vi "SV Time Waveforms State Manager.vi"(6 "delete hit index (-1 = last)":i32=-1, 7 "action":u16(ring)=3 items=["Initialize to Empty", "Add to State", "Delete from State", "Get Identifiers", "Get State"], 9 "1D Array of Current Time Data\n[reference, response0..N]":waveform(dbl)[](array[waveform]), 10 "Array of Node IDentifiers\n[reference{node, dir}, response0{node, dir}, ...]":T2(array[cluster]) {"active node" format="%04.0f"}, 11 "Time-Domain State":T3 {"IDentifiers"."Array of Node IDentifiers[reference{node, dir}, response0{node, dir}, ...]"."active node" format="%04.0f"}) -> (1 "2D Array of Time Data\n[[reference, response0..N] by [hit0..K]]":waveform(dbl)[][](array[waveform]), 2 "IDentifiers":T1(array[cluster]) {"Array of Node IDentifiers[reference{node, dir}, response0{node, dir}, ...]"."active node" format="%04.0f"}, 3 "Time-Domain State out":T3 {"IDentifiers"."Array of Node IDentifiers[reference{node, dir}, response0{node, dir}, ...]"."active node" format="%04.0f"}, 4 "number of impacts":i32[](array[numeric]), 5 "state changed":bool)   [LabVIEW 2017]
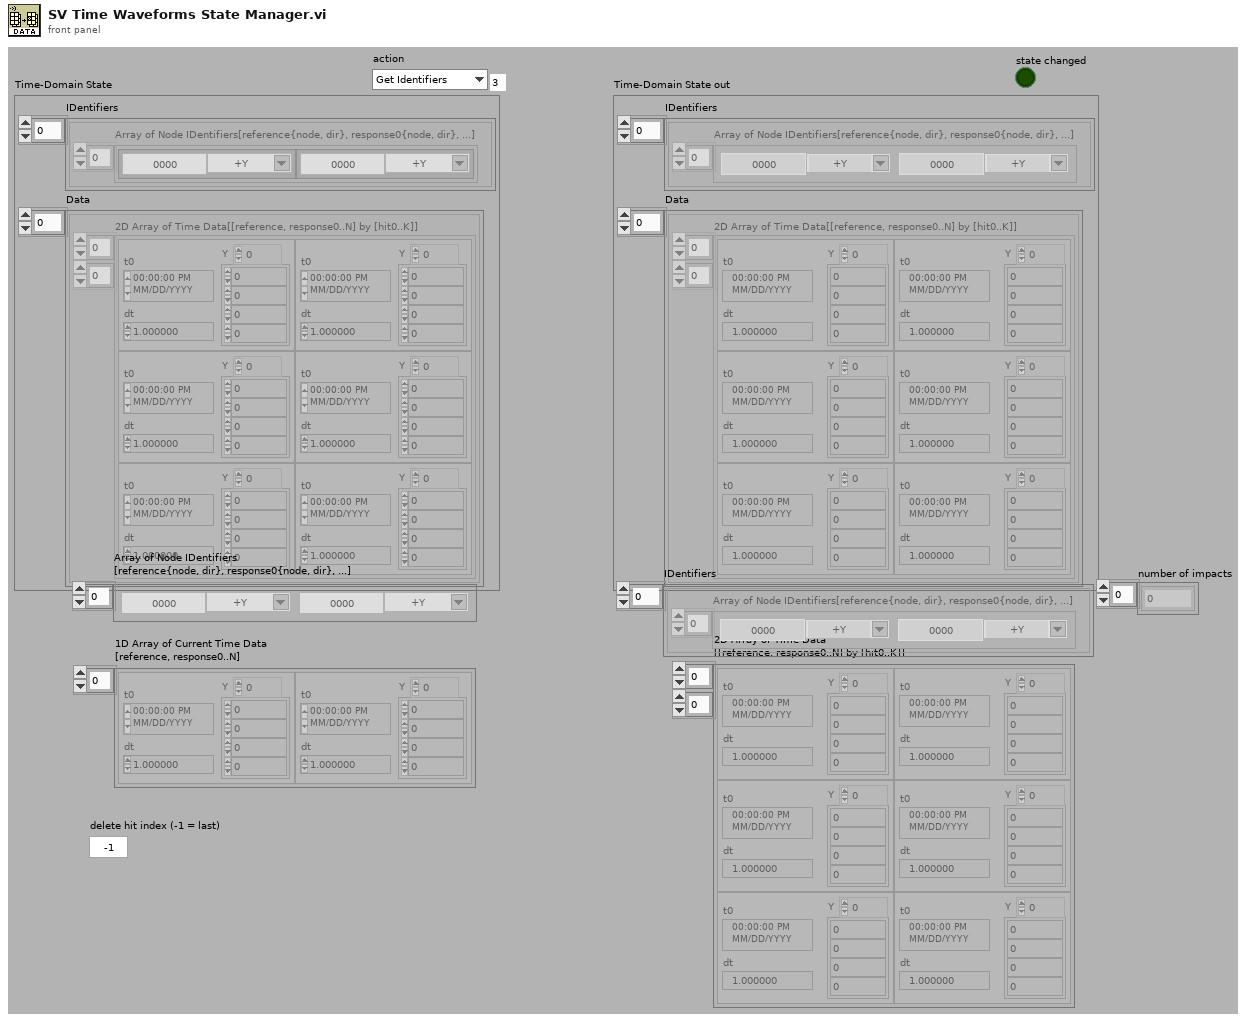
[diagram p1: front panel]
types:
  T1 = cluster{"Array of Node IDentifiers[reference{node, dir}, response0{node, dir}, ...]":cluster{"active node":i32, "coordinate":string}[]}[]
  T2 = cluster{"active node":i32, "coordinate":string}[]
  T3 = cluster{"IDentifiers":cluster{"Array of Node IDentifiers[reference{node, dir}, response0{node, dir}, ...]":cluster{"active node":i32, "coordinate":string}[]}[], "Data":cluster{"2D Array of Time Data[[reference, response0..N] by [hit0..K]]":waveform(dbl)[][]}[]}
  T4 = cluster{"2D Array of Time Data[[reference, response0..N] by [hit0..K]]":waveform(dbl)[][]}[]
  T5 = cluster{"2D Array of Time Data[[reference, response0..N] by [hit0..K]]":waveform(dbl)[][]}
  T6 = cluster{"Array of Node IDentifiers\n[reference{node, dir}, response0{node, dir}, ...]":cluster{"active node":i32, "coordinate":string}[]}
  T7 = cluster{"Array of Node IDentifiers\n[reference{node, dir}, response0{node, dir}, ...]":cluster{"active node":i32, "coordinate":string}[]}[]
  T8 = cluster{"Array of Node IDentifiers[reference{node, dir}, response0{node, dir}, ...]":cluster{"active node":i32, "coordinate":string}[]}
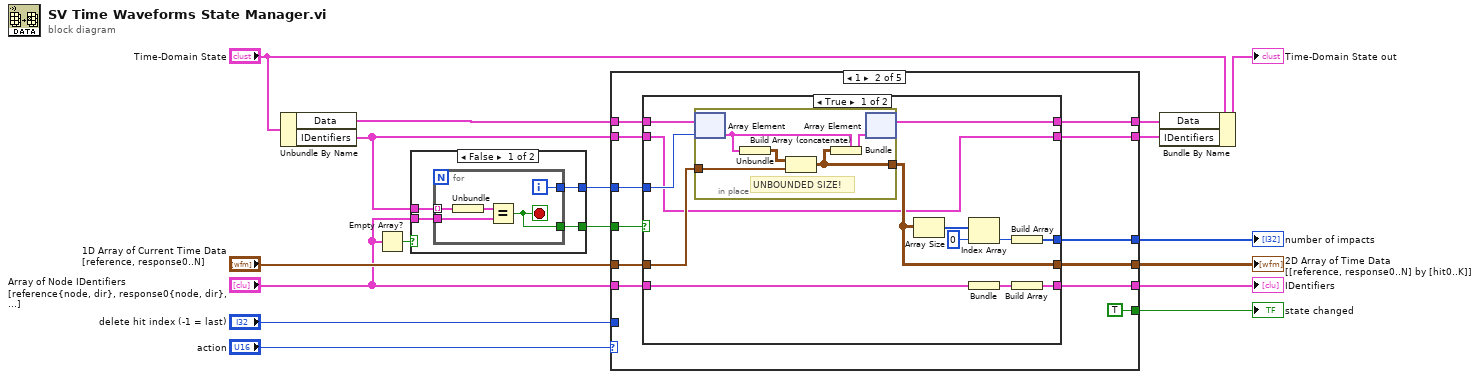
[diagram p0: block diagram]
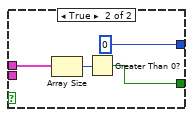
[diagram p2: hidden frame]
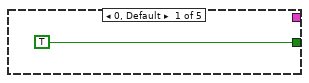
[diagram p3: hidden frame]
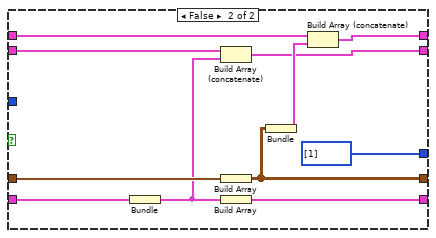
[diagram p4: hidden frame]
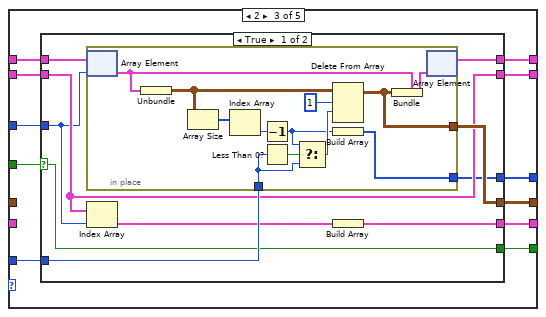
[diagram p5: hidden frame]
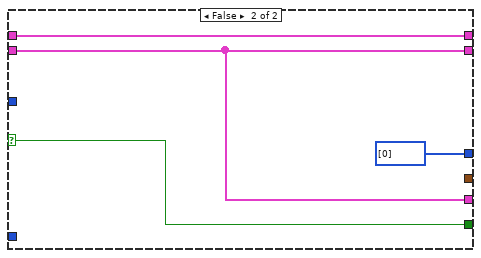
[diagram p6: hidden frame]
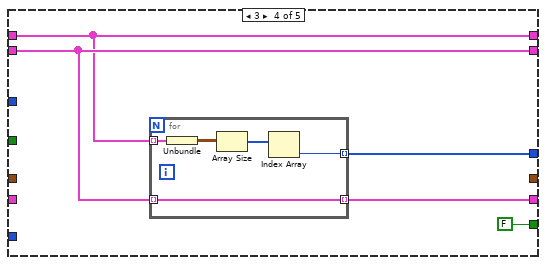
[diagram p7: hidden frame]
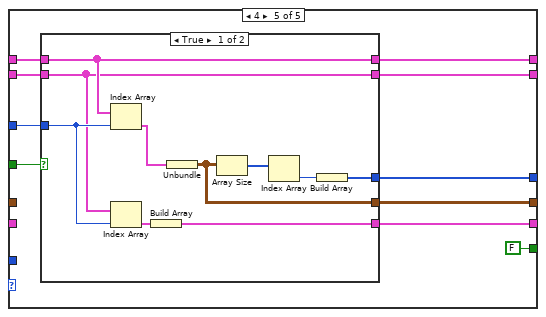
[diagram p8: hidden frame]
diagram:
  n1 = Unbundle By Name("Time-Domain State") -> ("Data"=w11:T4, "IDentifiers"=w8:T1)
  n2 = Empty Array?(array="Array of Node IDentifiers\n[reference{node, dir}, response0{node, dir}, ...]") -> (empty?=w7:bool)
  n3 = case shown="False" w7 {
    tunnel: [w21 0] -> w12
    tunnel: w8 -> [w20 w29]
    tunnel: [w19 w27] -> w4
    tunnel: "Array of Node IDentifiers\n[reference{node, dir}, response0{node, dir}, ...]" -> [w18 _]
    frame False {
      n4 = for {
        tunnel: w20 -> [w26] mode=indexing
        tunnel: w18 -> [w24]
        tunnel: [w23] -> w21
        tunnel: [w22] -> w19
        i -> [w23]
        stop <- w22 stop-if-true
        n5 = Unbundle(w26) -> ("Array of Node IDentifiers[reference{node, dir}, response0{node, dir}, ...]"=w25:T2)
        n6 = Equal?(x=w25, y=w24) -> (x = y?=w22:bool)
      }
    }
    frame True {
      n7 = Array Size(array=w29) -> (size(s)=w28:i32)
      n8 = Greater Than 0?(x=w28) -> (x > 0?=w27:bool)
    }
  }
  n9 = case shown="1" "action" {
    tunnel: "Array of Node IDentifiers\n[reference{node, dir}, response0{node, dir}, ...]" -> [_ w43 _ _ _]
    tunnel: "1D Array of Current Time Data\n[reference, response0..N]" -> [_ w42 _ _ _]
    tunnel: "delete hit index (-1 = last)" -> [_ _ w83 _ _]
    tunnel: [_ w34 w82 w111 w129] -> w14
    tunnel: [_ w41 w81 _ w128] -> w13
    tunnel: w12 -> [_ w38 w79 _ w127]
    tunnel: w11 -> [_ w40 w80 w112 w126]
    tunnel: [_ w37 w78 w112 w125] -> w9
    tunnel: w8 -> [_ w39 w75 w113 w124]
    tunnel: [_ w35 w73 w113 w123] -> w6
    tunnel: w4 -> [_ w36 w77 _ w122]
    tunnel: [TRUE TRUE w76 FALSE FALSE] -> w3
    tunnel: [_ w32 w74 w110 w120] -> w1
    frame 0, Default {
    }
    frame 1 {
      n10 = case shown="True" w36 {
        tunnel: w40 -> [w47 w71]
        tunnel: w38 -> [w46 _]
        tunnel: w42 -> [w56 w70]
        tunnel: w39 -> [w44 w68]
        tunnel: w43 -> [w55 w69]
        tunnel: [w45 w67] -> w37
        tunnel: [w44 w66] -> w35
        tunnel: [w51 w65] -> w41
        tunnel: [w53 w63] -> w34
        tunnel: [w48 i32[] [1]] -> w32
        frame True {
          n11 = in-place {
            in-place-border: w56 -> [w60]
            in-place-border: [w57] -> w51
            # "UNBOUNDED SIZE!"
            n12 = in-place-array #1(w47, w46) -> (w59:T5)
            n13 = Unbundle(w59) -> ("2D Array of Time Data[[reference, response0..N] by [hit0..K]]"=w61:waveform(dbl)[][])
            n14 = Build Array (concatenate)(w61, w60) -> (w57:waveform(dbl)[][])
            n15 = Bundle(cluster=w59, "2D Array of Time Data[[reference, response0..N] by [hit0..K]]"=w57) -> (w58:T5)
            n16 = in-place-array #1(w58) -> (w45:T4)  [unwired: 1 out]
          }
          n17 = Array Size(array=w51) -> (size(s)=w52:i32[])
          n18 = Index Array(array=w52, index=0) -> (element=w49:i32)
          n19 = Bundle("Array of Node IDentifiers\n[reference{node, dir}, response0{node, dir}, ...]"=w55) -> (w54:T6)  [unwired: 1 in]
          n20 = Build Array(w49) -> (w48:i32[])
          n21 = Build Array(w54) -> (w53:T7)
        }
        frame False {
          n22 = Bundle("Array of Node IDentifiers\n[reference{node, dir}, response0{node, dir}, ...]"=w69) -> (w64:T6)  [unwired: 1 in]
          n23 = Build Array (concatenate)(w68, w64) -> (w66:T7)
          n24 = Build Array(w70) -> (w65:waveform(dbl)[][])
          n25 = Build Array(w64) -> (w63:T7)
          n26 = Bundle(w65) -> (w72:cluster{waveform(dbl)[][]})  [unwired: 1 in]
          n27 = Build Array (concatenate)(w71, w72) -> (w67:T4)
        }
      }
    }
    frame 2 {
      n28 = case shown="True" w77 {
        selector: w77 -> [w89 w108]
        tunnel: w80 -> [w87 w109]
        tunnel: w79 -> [w85 _]
        tunnel: w75 -> [w88 w106]
        tunnel: [w86 w109] -> w78
        tunnel: [w90 w106] -> w82
        tunnel: w83 -> [w93 _]
        tunnel: [w92 _] -> w81
        tunnel: [w89 w108] -> w76
        tunnel: [w84 i32[] [0]] -> w74
        tunnel: [w88 w106] -> w73
        frame True {
          n29 = in-place {
            in-place-border: w93 -> [w100]
            in-place-border: [w96] -> w92
            in-place-border: [w94] -> w84
            n30 = in-place-array #2(w87, w85) -> (w98:T5)
            n31 = Unbundle(w98) -> ("2D Array of Time Data[[reference, response0..N] by [hit0..K]]"=w99:waveform(dbl)[][])
            n32 = Array Size(array=w99) -> (size(s)=w102:i32[])
            n33 = Index Array(array=w102) -> (element=w101:i32)  [unwired: 1 in]
            n34 = Decrement(x=w101) -> (x-1=w95:i32)
            n35 = Less Than 0?(x=w100) -> (x < 0?=w104:bool)
            n36 = Select(t=w95, s=w104, f=w100) -> (s? t:f=w103:i32)
            n37 = Delete From Array(array=w99, length=1, index (row)=w103) -> (array with subset deleted=w96:waveform(dbl)[][])  [unwired: 1 in, 1 out]
            n38 = Build Array(w95) -> (w94:i32[])
            n39 = Bundle(cluster=w98, "2D Array of Time Data[[reference, response0..N] by [hit0..K]]"=w96) -> (w97:T5)
            n40 = in-place-array #2(w97) -> (w86:T4)  [unwired: 1 out]
          }
          n41 = Index Array(array=w88, index=w85) -> (element=w91:T8)
          n42 = Build Array(w91) -> (w90:T1)
        }
        frame False {
        }
      }
    }
    frame 3 {
      n43 = for {
        tunnel: w113 -> [w119] mode=indexing
        tunnel: w112 -> [w118] mode=indexing
        tunnel: [w119] -> w111 mode=indexing
        tunnel: [w115] -> w110 mode=indexing
        n44 = Unbundle(w118) -> ("2D Array of Time Data[[reference, response0..N] by [hit0..K]]"=w117:waveform(dbl)[][])
        n45 = Array Size(array=w117) -> (size(s)=w116:i32[])
        n46 = Index Array(array=w116) -> (element=w115:i32)  [unwired: 1 in]
      }
    }
    frame 4 {
      n47 = case shown="True" w122 {
        tunnel: w126 -> [w138 w141]
        tunnel: w127 -> [w136 _]
        tunnel: w124 -> [w134 w140]
        tunnel: [w138 w141] -> w125
        tunnel: [w135 _] -> w129
        tunnel: [w132 _] -> w128
        tunnel: [w134 w140] -> w123
        tunnel: [w130 _] -> w120
        frame True {
          n48 = Index Array(array=w138, index=w136) -> (element=w139:T5)
          n49 = Index Array(array=w134, index=w136) -> (element=w137:T8)
          n50 = Build Array(w137) -> (w135:T1)
          n51 = Unbundle(w139) -> ("2D Array of Time Data[[reference, response0..N] by [hit0..K]]"=w132:waveform(dbl)[][])
          n52 = Array Size(array=w132) -> (size(s)=w133:i32[])
          n53 = Index Array(array=w133) -> (element=w131:i32)  [unwired: 1 in]
          n54 = Build Array(w131) -> (w130:i32[])
        }
        frame False {
        }
      }
    }
  }
  "2D Array of Time Data\n[[reference, response0..N] by [hit0..K]]" <- w13
  "IDentifiers" <- w14
  "state changed" <- w3
  "number of impacts" <- w1
  n55 = Bundle By Name(cluster="Time-Domain State", "Data"=w9, "IDentifiers"=w6) -> (→"Time-Domain State out":T3)
